vi "Get Object Type.vi"(8 "Error In":errorcluster, 11 "reference in":refnum<class "OD Entry.lvclass">) -> (0 "Error Out":errorcluster, 1 "Defined?":bool, 2 "ObjectType":T1 items=["NULL"=0, "DOMAIN"=2, "DEFTYPE"=5, "DEFSTRUCT"=6, "VAR"=7, "ARRAY"=8, "RECORD"=9], 3 "reference out":refnum<class "OD Entry.lvclass">)   [LabVIEW 2024, in "EDS.lvlib" / "OD Entry.lvclass"]
uses:
  OD Entry.lvclass
  Object Type.ctl
  Object Type/Object Type Base.lvclass
  OD Entry.lvclass/OD Entry.ctl
  EDS.lvlib
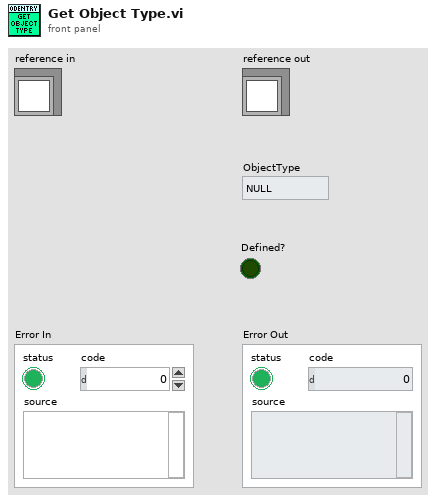
[diagram p1: front panel]
types:
  T1 = typedef "EDS.lvlib/Object Type.ctl" = u8
  T2 = typedef "EDS.lvlib/OD Entry.lvclass/ObjectAttributes.ctl" = cluster{"Index":u16, "Object Type":refnum<class "Object Type Base.lvclass">, "Denotation":string, "Count":u8, "ObjExtend":u8, "PDOtype":T3, "Label":string, "Description":string, "Sub-Entries":map{u16, refnum<class "OD Sub-Entry.lvclass">}}
  T3 = typedef "EDS.lvlib/PDO Mapping Type.ctl" = enum16{"NO", "OPTIONAL", "RPDO", "TPDO", "DEFAULT"}
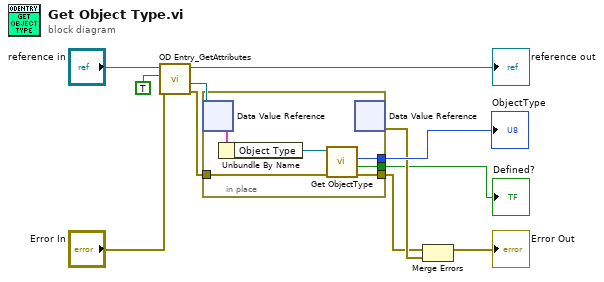
[diagram p0: block diagram]
diagram:
  n1 = call "OD Entry_GetAttributes.vi"("Error In"="Error In", "OnlyGetDvrReference(False)"=TRUE, "reference in"="reference in") -> ("Error Out"=w3:errorcluster, "DataRef"=w4:refnum<data-value>, "reference out"=→"reference out":refnum<class "OD Entry.lvclass">)  [unwired: 5 in, 1 out]
  n2 = in-place {
    in-place-border: w3 -> [w15]
    in-place-border: [w14] -> w2
    in-place-border: [w13] -> w7
    in-place-border: [w12] -> w1
    n3 = in-place-dvr #1(w4) -> (w16:T2)  [unwired: 1 out]
    n4 = Unbundle By Name(w16) -> ("Object Type"=w17:refnum<class "Object Type Base.lvclass">)
    n5 = call-dynamic "Get ObjectType.vi"("error in"=w15, "Object Type in"=w17) -> ("error out"=w14:errorcluster, "Defined?"=w12:bool, "ObjectType"=w13:T1)  [unwired: 6 in, 1 out]
    n6 = in-place-dvr #1() -> (w6:errorcluster)  [unwired: 1 in, 1 out]
  }
  "ObjectType" <- w7
  "Defined?" <- w1
  n7 = Merge Errors(w2, w6) -> (→"Error Out":errorcluster)
